vi "Read Unlock Publication Msg.vi"(11 "IModel in":refnum<class "IModel.lvclass">) -> (2 "Pre-Addressed Unlock Msg":refnum<class "Unlock Publication Msg.lvclass">)   [LabVIEW 2017, in "IModel.lvlib" / "IModel.lvclass"]
uses:
  <vilib>/gpm_packages/@cs/mva-core/Source/IModel/IModel/IModel.lvclass
  <vilib>/gpm_packages/@cs/mva-core/Source/IMediator/IMediator Messages/Unlock Publication Msg/Unlock Publication Msg.lvclass
  <vilib>/gpm_packages/@cs/mva-core/Source/IModel/IModel/IModel.lvclass/IModel.ctl
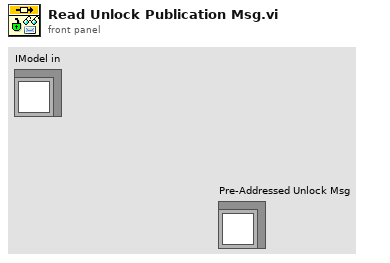
[diagram p1: front panel]
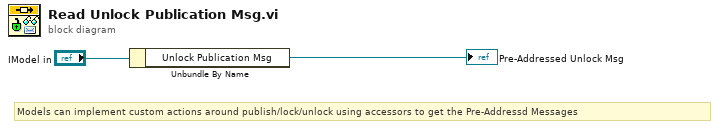
[diagram p0: block diagram]
diagram:
  # "Models can implement custom actions around publish/lock/unlock using accessors to get the Pre-Addressd Messages"
  n1 = Unbundle By Name("IModel in") -> ("Unlock Publication Msg"=→"Pre-Addressed Unlock Msg":refnum<class "Unlock Publication Msg.lvclass">)
